vi "Data Viewer.vi"() -> ()   [LabVIEW 2015]
uses:
  Libraries/File/Controls/Data Viewer Entry.ctl
  Libraries/File/Controls/Channel name entry.ctl
  Libraries/File/Controls/Data reduction.ctl
panel:
  in  "Relative time":bool
  out "Dy":dbl format="%#_4p"
  out "1/Dx":dbl format="%#_4p"
  out "Dx":dbl format="%#_4p"
  in  "Decimation method":T1(ring)=enum."Min-Max"
  in  "Max points (-1:all)":i32=1000000 format="%.0p"
  in  "Clip time":bool
  in  "Time interval":cluster{dbl, dbl}(slide)={0.1, -0.01} scale=-0.01..0.1 scale format="%#_6p"
  in  "Clear all":bool
  in  "stop":bool
  out "XY Graph":cluster{dbl[], dbl[]}[](graph)
  in  "Group name":string="Untitled"
  in  "Data files":T2[](array[typedef])
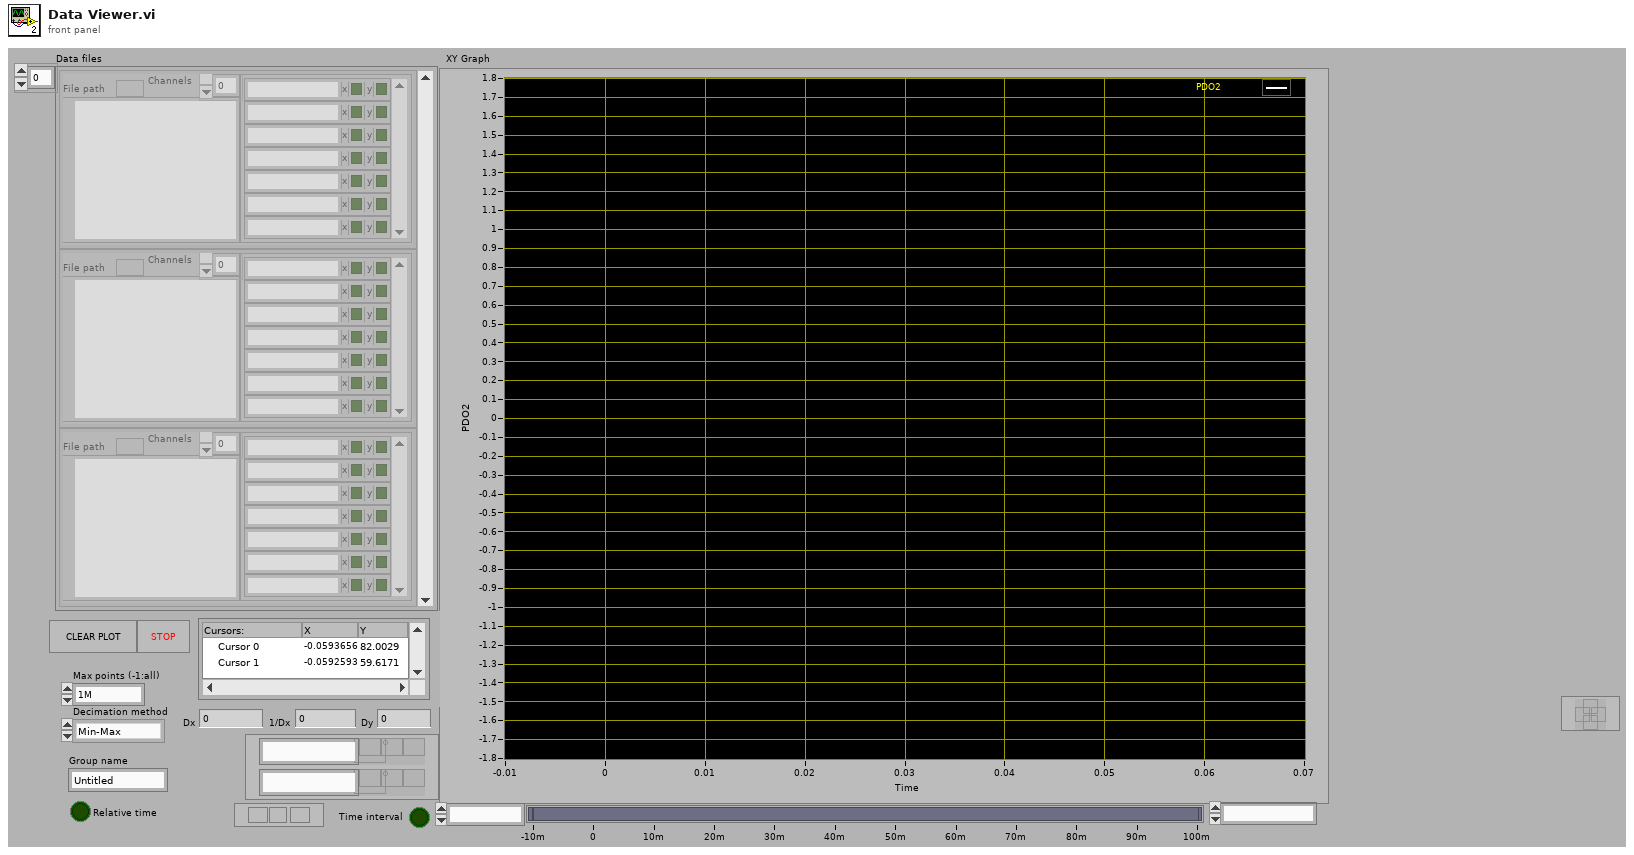
[diagram p1: front panel]
types:
  T1 = enum16{"coerce", "linear", "spline", "Min-Max", "Average"}
  T2 = typedef "Data Viewer Entry.ctl" = cluster{"File path":path, "Channels":T3[]}
  T3 = typedef "Channel name entry.ctl" = cluster{"Name":string, "x":bool, "y":bool}
  T4 = typedef "Data reduction.ctl" = cluster{"Clip time":bool, "Tiime 0":dbl, "Time 1":dbl, "Maximum data points":i32, "Decimation method":enum16{"coerce", "linear", "spline", "Min-Max", "Average"}}
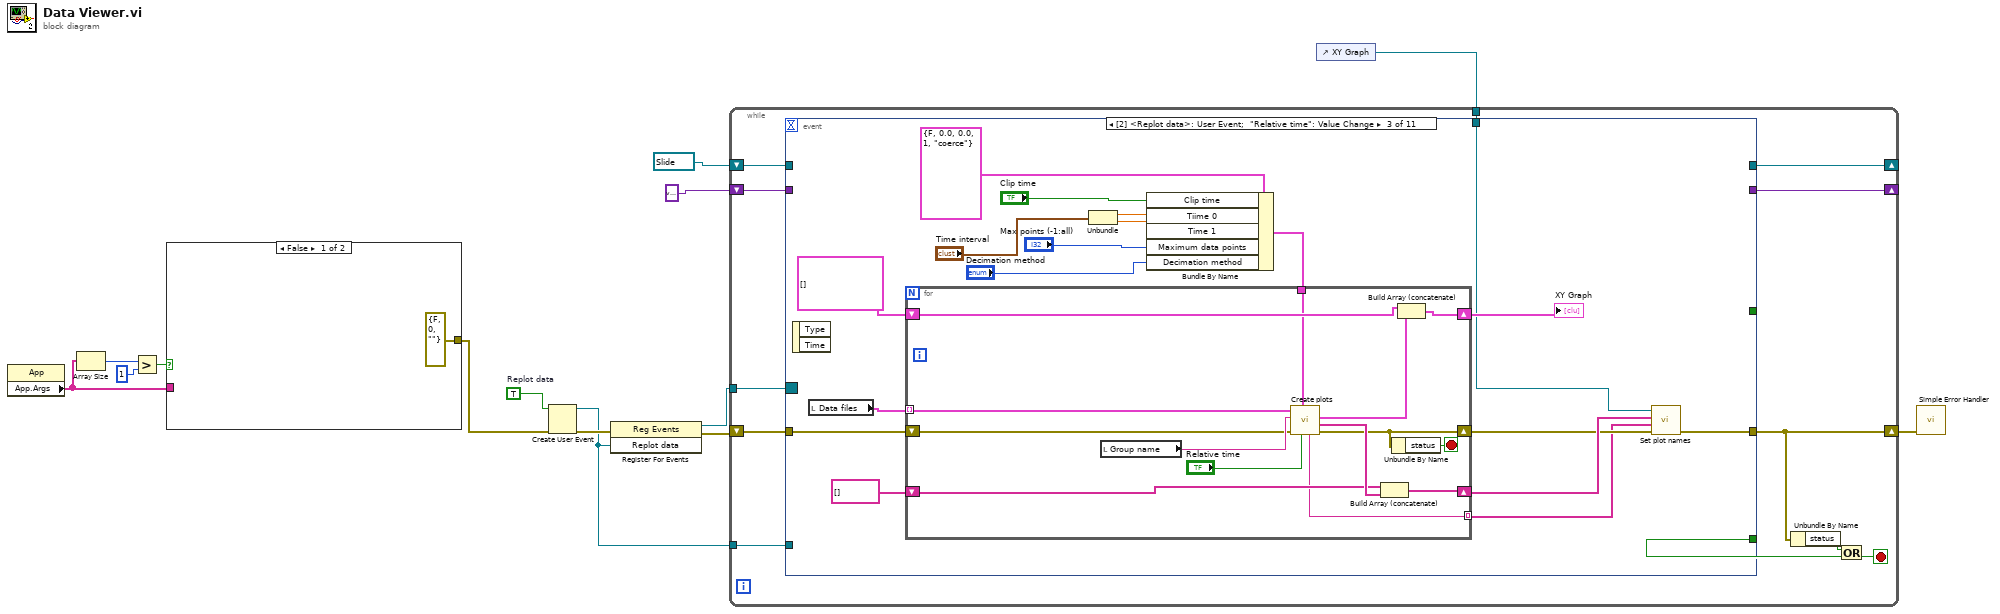
[diagram p0: block diagram]
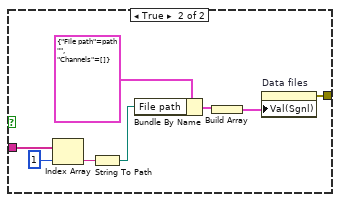
[diagram p2: hidden frame]
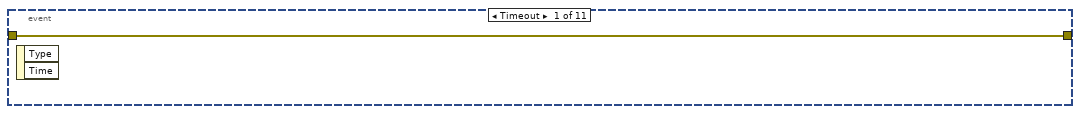
[diagram p3: hidden frame]
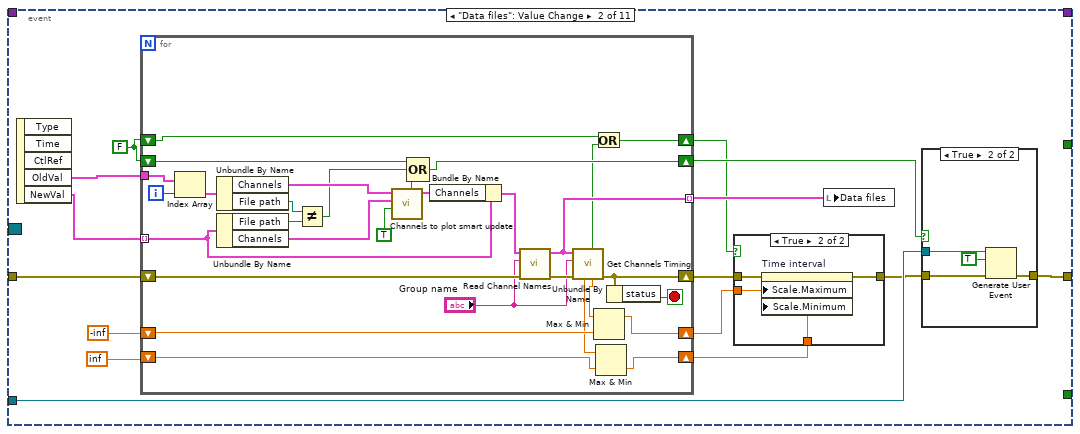
[diagram p4: hidden frame]
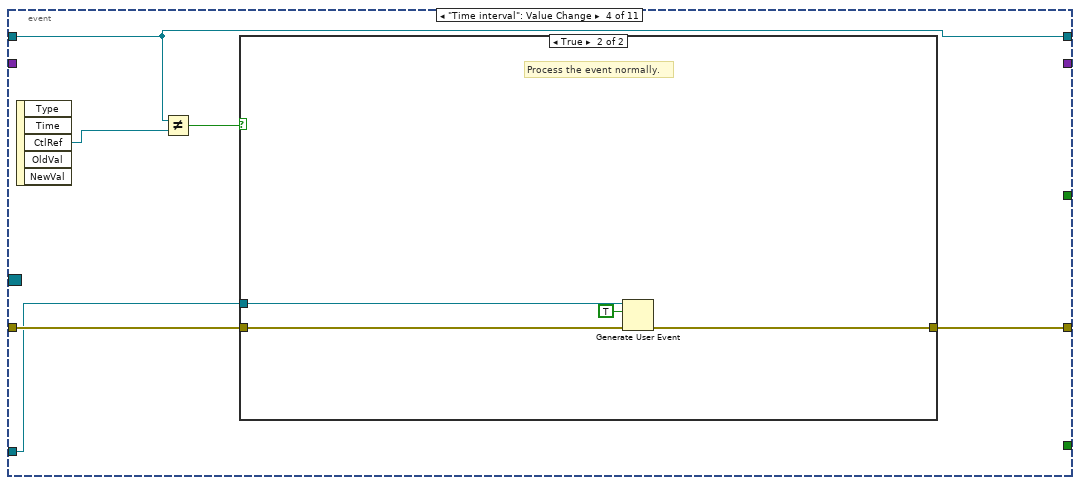
[diagram p7: hidden frame]
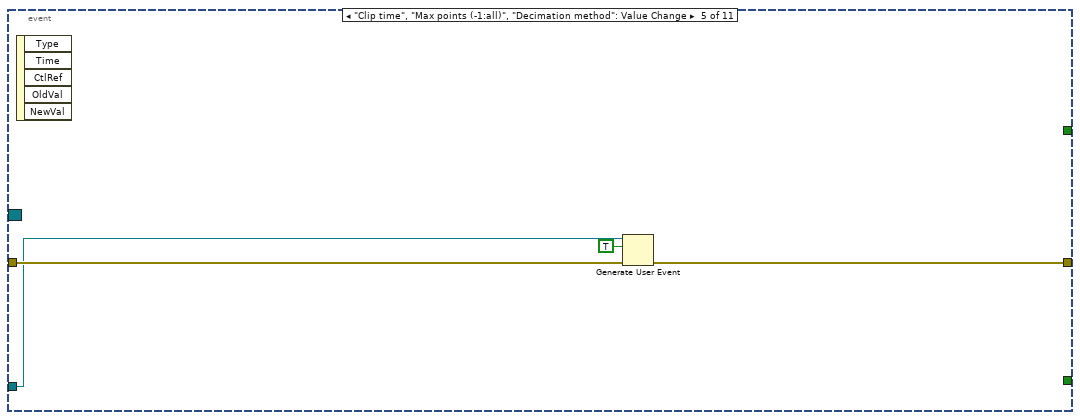
[diagram p9: hidden frame]
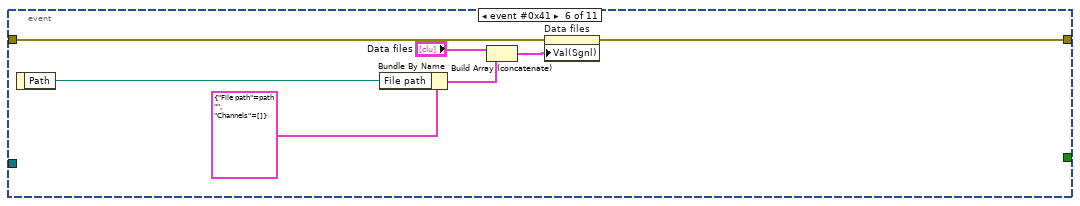
[diagram p10: hidden frame]
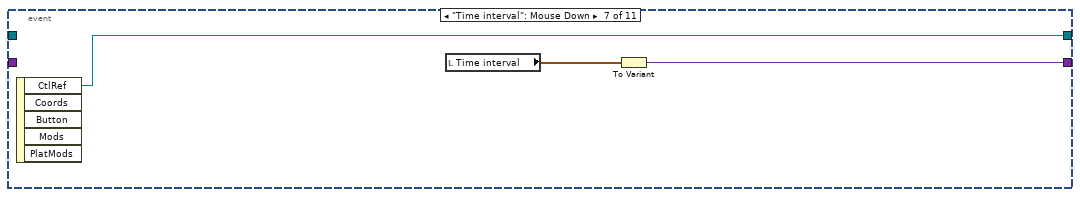
[diagram p11: hidden frame]
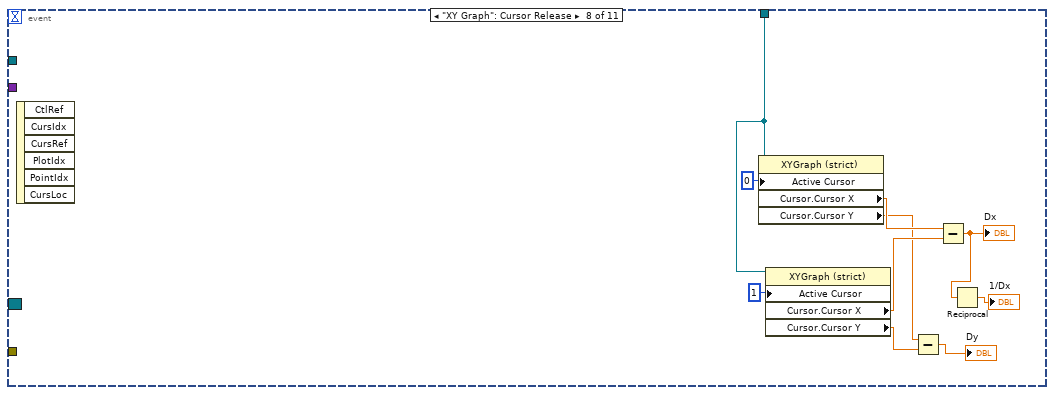
[diagram p12: hidden frame]
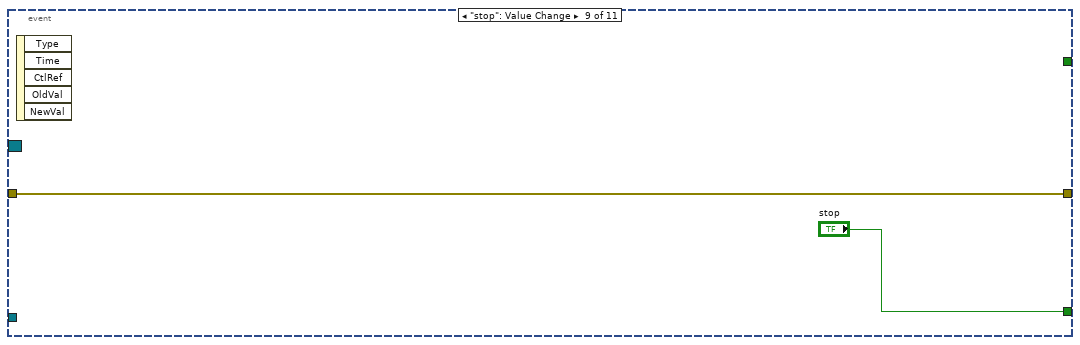
[diagram p13: hidden frame]
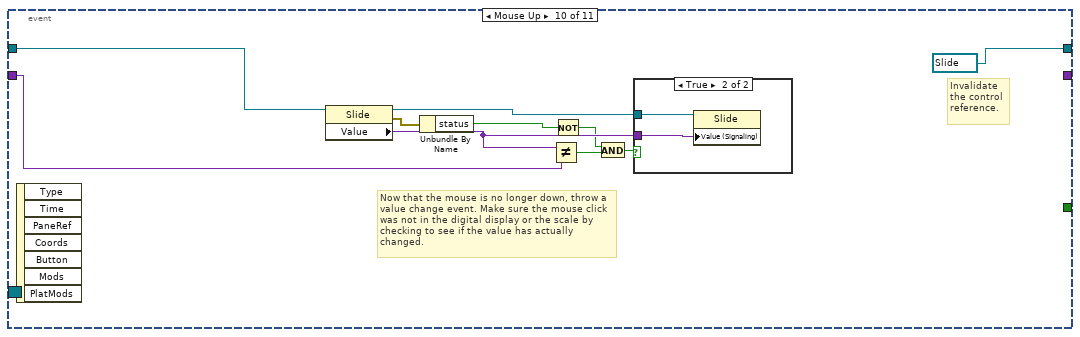
[diagram p14: hidden frame]
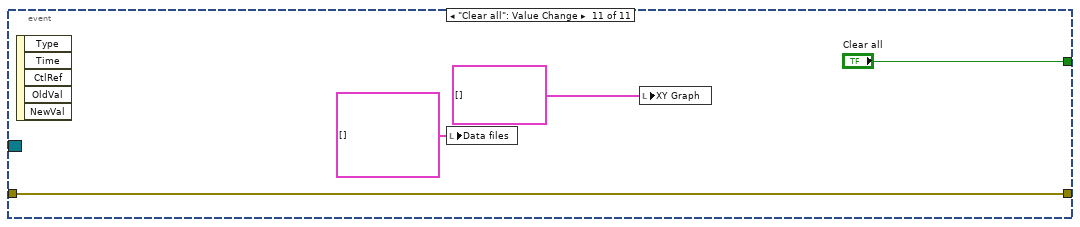
[diagram p16: hidden frame]
diagram:
  w9 = TRUE  # Replot data
  n1 = property class="App"() -> ("App.Args"=w13:string[])  [unwired: 2 in, 2 out]
  n2 = Array Size(array=w13) -> (size(s)=w12:i32)
  n3 = Greater?(x=w12, y=1) -> (0:w10:bool)
  n4 = case shown="False" w10 {
    tunnel: w13 -> [_ w23]
    tunnel: [errorcluster {"status"=FALSE, "code"=0, "source"=""} ("error out") w16] -> w7
    frame False {
    }
    frame True {
      n5 = Index Array(array=w23, index=1) -> (element=w21:string)
      n6 = String To Path(string=w21) -> (path=w19:path)
      n7 = Bundle By Name(cluster=T2 {"File path"=path "", "Channels"=[]} ("Cluster"), "File path"=w19) -> (w18:T2)
      n8 = Build Array(w18) -> (w17:T2[])
      n9 = property on="Data files" class="Arr (strict)"("Val(Sgnl)"=w17) -> (error out=w16:errorcluster)  [unwired: 2 in, 1 out]
    }
  }
  n10 = Create User Event(user event datatype=w9, error in=w7) -> (user event=w4:refnum<user-event>, error out=w8:errorcluster)
  n11 = register-events(error in=w8, w4) -> (reference out=w5:refnum<event-registration>, error out=w6:errorcluster)  [unwired: 1 in]
  n12 = control-ref of="XY Graph"() -> (w1:refnum<vi>)
  n13 = while {
    shift-right: [w31] -> w14
    shift-left: w6 -> [w35]
    tunnel: w5 -> [w30]
    tunnel: w4 -> [w29]
    shift-right: [w25] -> _
    shift-left: refnum<vi> refnum ("CtlRef") -> [w28]
    shift-right: [w26] -> _
    shift-left: variant ("Variant") -> [w27]
    tunnel: w1 -> [w24]
    stop <- w33 stop-if-true
    n14 = event shown="[2] <Replot data>: User Event;  \"Relative time\": Value Change" {
      selector: w30 -> [_ _ _ _ _ _ _ _ _ _ _]
      dyn-events: _ -> [_ _ _ _ _ _ _ _ _ _ _]
      timeout: _ -> [_ _ _ _ _ _ _ _ _ _ _]
      tunnel: w35 -> [w36 w50 w109 w126 w138 w140 _ _ w160 _ w175]
      tunnel: [w36 w47 w106 w125 w137 w139 _ _ w160 _ w175] -> w31
      tunnel: [_ _ _ _ _ _ _ _ "stop" _ _] -> w34
      tunnel: [_ _ _ _ _ _ _ _ _ _ "Clear all"] -> _
      tunnel: w29 -> [_ w48 _ w124 w136 _ _ _ _ _ _]
      tunnel: w28 -> [_ _ _ w127 _ _ _ _ _ w163 _]
      tunnel: w27 -> [_ _ _ _ _ _ _ _ _ w162 _]
      tunnel: [_ _ _ _ _ _ w147 _ _ _ _] -> w26
      tunnel: [_ _ _ w127 _ _ w146 _ _ refnum<vi> refnum ("CtlRef") _] -> w25
      tunnel: w24 -> [_ _ w92 _ _ _ _ w157 _ _ _]
      event Timeout {
        n15 = event-data() -> ()  [unwired: 1 in, 2 out]
      }
      event "Data files": Value Change {
        w38 = FALSE
        n16 = event-data() -> ("OldVal"=w49:T2[], "NewVal"=w51:T2[])  [unwired: 1 in, 3 out]
        n17 = for {
          tunnel: w51 -> [w84] mode=indexing
          shift-right: [w75] -> w42
          shift-left: w50 -> [w85]
          tunnel: w49 -> [w89]
          tunnel: [w77] -> w45 mode=indexing
          shift-right: [w78] -> w46
          shift-left: w38 -> [w79]
          shift-right: [w72] -> w40
          shift-left: -inf -> [w73]
          shift-right: [w71] -> w39
          shift-left: inf -> [w69]
          shift-right: [w65] -> w37
          shift-left: w38 -> [w67]
          i -> [w88]
          stop <- w91 stop-if-true
          n18 = Index Array(array=w89, index=w88) -> (element=w87:T2)
          n19 = Unbundle By Name(w87) -> ("Channels"=w86:T3[], "File path"=w64:path)
          n20 = Unbundle By Name(w84) -> ("File path"=w63:path, "Channels"=w90:T3[])
          n21 = Not Equal?(x=w64, y=w63) -> (x != y?=w62:bool)
          n22 = call "Channels to plot smart update.vi"("Disable y for 1st channel"=TRUE, "Channels to plot new value"=w90, "Channels to plot old value"=w86) -> ("Channels to plot out"=w83:T3[], "Replot?"=w80:bool)  [unwired: 1 in, 6 out]
          n23 = Compound Arithmetic op=OR(w79, w62, w80) -> (w78:bool)
          n24 = Bundle By Name(cluster=w84, "Channels"=w83) -> (w82:T2)
          n25 = call "Read Channel Names.vi"("error in"=w85, "group name"="Group name", "Data record"=w82) -> ("error out"=w76:errorcluster, "Data record out"=w77:T2)  [unwired: 7 in]
          n26 = call "Get Channels Timing.vi"("error in (no error)"=w76, "group name in"="Group name", "Data file"=w77) -> ("error out"=w75:errorcluster, "Latest finish"=w74:dbl, "Plots exist"=w66:bool, "Earliest start"=w70:dbl)  [unwired: 4 in, 1 out]
          n27 = Or(x=w67, y=w66) -> (x .or. y?=w65:bool)
          n28 = Max & Min(x=w74, y=w73) -> (max(x,y)=w72:dbl)  [unwired: 1 out]
          n29 = Max & Min(x=w70, y=w69) -> (min(x,y)=w71:dbl)  [unwired: 1 out]
          n30 = Unbundle By Name(w75) -> ("status"=w91:bool)
        }
        n31 = case shown="True" w37 {
          tunnel: w42 -> [w52 w56]
          tunnel: [w52 w55] -> w41
          tunnel: w40 -> [_ w54]
          tunnel: w39 -> [_ w53]
          frame False {
          }
          frame True {
            n32 = property on="Time interval" class="Slide (strict)"(error in=w56, "Scale.Maximum"=w54, "Scale.Minimum"=w53) -> (error out=w55:errorcluster)  [unwired: 1 in, 1 out]
          }
        }
        n33 = local write "Data files"(w45) -> ()
        n34 = case shown="True" w46 {
          tunnel: w48 -> [_ w61]
          tunnel: w41 -> [w57 w60]
          tunnel: [w57 w59] -> w47
          frame False {
          }
          frame True {
            n35 = Generate User Event(user event=w61, event data cluster=TRUE ("event data"), error in=w60) -> (error out=w59:errorcluster)  [unwired: 1 in, 1 out]
          }
        }
      }
      event User Event; "Relative time": Value Change {
        n36 = event-data() -> ()  [unwired: 1 in, 2 out]
        n37 = local read "Data files"() -> (w102:T2[])
        n38 = Unbundle("Time interval") -> (w97:dbl, w96:dbl)
        n39 = Bundle By Name(cluster=T4 {"Clip time"=FALSE, "Tiime 0"=0.0, "Time 1"=0.0, "Maximum data points"=1, "Decimation method"=enum."coerce"} ("Data reduction"), "Clip time"="Clip time", "Tiime 0"=w97, "Time 1"=w96, "Maximum data points"="Max points (-1:all)", "Decimation method"="Decimation method") -> (w95:T4)
        n40 = for {
          shift-right: [w119] -> w105
          shift-left: w109 -> [w112]
          shift-right: [w121] -> w107
          shift-left: string[] [] -> [w120]
          shift-right: [w117] -> w101
          shift-left: cluster{sgl[], sgl[]}[] [] -> [w116]
          tunnel: [w115] -> w103 mode=indexing
          tunnel: w102 -> [w114] mode=indexing
          tunnel: w95 -> [w111]
          stop <- w123 stop-if-true
          n41 = local read "Group name"() -> (w113:string)
          n42 = call "Create plots.vi"("Relative time"="Relative time", "Data reduction"=w111, "error in (no error)"=w112, "group name in"=w113, "Data record"=w114) -> ("error out"=w119:errorcluster, "Y names"=w122:string[], "Plots"=w118:cluster{dbl[], dbl[]}[], "X-axis name"=w115:string)  [unwired: 2 in, 1 out]
          n43 = Build Array (concatenate)(w120, w122) -> (w121:string[])
          n44 = Unbundle By Name(w119) -> ("status"=w123:bool)
          n45 = Build Array (concatenate)(w116, w118) -> (w117:cluster{dbl[], dbl[]}[])
        }
        "XY Graph" <- w101
        n46 = call "Set plot names.vi"("error in"=w105, "X-axis names"=w103, "Plot names"=w107, "XYGraph Refnum"=w92) -> ("error out"=w106:errorcluster)  [unwired: 6 in, 1 out]
      }
      event "Time interval": Value Change {
        n47 = event-data() -> ("CtlRef"=w129:refnum<vi>)  [unwired: 1 in, 4 out]
        n48 = Not Equal?(x=w127, y=w129) -> (x != y?=w128:bool)
        n49 = case shown="True" w128 {
          tunnel: w126 -> [w130 w133]
          tunnel: [w130 w132] -> w125
          tunnel: w124 -> [_ w131]
          frame False {
            # "Value changed, but the mouse button is still down, so disregard the event."
          }
          frame True {
            # "Process the event normally."
            n50 = Generate User Event(user event=w131, event data cluster=TRUE ("event data"), error in=w133) -> (error out=w132:errorcluster)  [unwired: 1 in, 1 out]
          }
        }
      }
      event "Clip time", "Max points (-1:all)", "Decimation method": Value Change {
        n51 = event-data() -> ()  [unwired: 1 in, 5 out]
        n52 = Generate User Event(user event=w136, event data cluster=TRUE ("event data"), error in=w138) -> (error out=w137:errorcluster)  [unwired: 1 in, 1 out]
      }
      event event #0x41 {
        n53 = event-data() -> ("Path"=w143:path)  [unwired: 1 in]
        n54 = Bundle By Name(cluster=T2 {"File path"=path "", "Channels"=[]} ("Cluster"), "File path"=w143) -> (w145:T2)
        n55 = Build Array (concatenate)("Data files", w145) -> (w141:T2[])
        n56 = property on="Data files" class="Arr (strict)"(error in=w140, "Val(Sgnl)"=w141) -> (error out=w139:errorcluster)  [unwired: 1 in, 1 out]
      }
      event "Time interval": Mouse Down {
        n57 = event-data() -> ("CtlRef"=w146:refnum<vi>)  [unwired: 1 in, 4 out]
        n58 = local read "Time interval"() -> (w148:cluster{dbl, dbl})
        n59 = To Variant(anything=w148) -> (Variant=w147:variant)
      }
      event "XY Graph": Cursor Release {
        n60 = event-data() -> ()  [unwired: 1 in, 6 out]
        n61 = property class="XYGraph (strict)"(reference=w157, "Active Cursor"=0 ("Cursor.Cursor Index")) -> ("Cursor.Cursor X"=w155:dbl, "Cursor.Cursor Y"=w151:dbl)  [unwired: 1 in, 2 out]
        n62 = property class="XYGraph (strict)"(reference=w157, "Active Cursor"=1 ("Cursor.Cursor Index")) -> ("Cursor.Cursor X"=w154:dbl, "Cursor.Cursor Y"=w150:dbl)  [unwired: 1 in, 2 out]
        n63 = Subtract(x=w151, y=w150) -> (x-y=→"Dy":dbl)
        n64 = Subtract(x=w155, y=w154) -> (x-y=w152:dbl)
        "Dx" <- w152
        n65 = Reciprocal(x=w152) -> (1/x=→"1/Dx":dbl)
      }
      event "stop": Value Change {
        n66 = event-data() -> ()  [unwired: 1 in, 5 out]
      }
      event Mouse Up {
        # "Invalidate\nthe control\nreference."
        # "Now that the mouse is no longer down, throw a value change event. Make sure the mouse click was not in the digital display or the scale by checking to see if the value has actually changed."
        n67 = event-data() -> ()  [unwired: 1 in, 7 out]
        n68 = property class="Slide"(reference=w163) -> (reference out=w170:refnum<vi>, error out=w169:errorcluster, "Value"=w168:variant)  [unwired: 1 in]
        n69 = Unbundle By Name(w169) -> ("status"=w166:bool)
        n70 = Not Equal?(x=w168, y=w162) -> (x != y?=w167:bool)
        n71 = Not(x=w166) -> (.not. x?=w164:bool)
        n72 = And(x=w164, y=w167) -> (x .and. y?=w165:bool)
        n73 = case shown="True" w165 {
          tunnel: w168 -> [_ w172]
          tunnel: w170 -> [_ w171]
          frame False {
          }
          frame True {
            n74 = property class="Slide"(reference=w171, "Value (Signaling)"=w172) -> ()  [unwired: 1 in, 2 out]
          }
        }
      }
      event "Clear all": Value Change {
        n75 = event-data() -> ()  [unwired: 1 in, 5 out]
        n76 = local write "Data files"(T2[] [] ("Data files")) -> ()
        n77 = local write "XY Graph"(cluster{dbl[], dbl[]}[] [] ("XY Graph")) -> ()
      }
    }
    n78 = Unbundle By Name(w31) -> ("status"=w32:bool)
    n79 = Or(x=w32, y=w34) -> (x .or. y?=w33:bool)
  }
  n80 = call <vilib>:"Simple Error Handler.vi"("error in (no error)"=w14) -> ()  [unwired: 4 in, 5 out]
